vi "sub_rplidar_check.vi"(8 "error in (no error)":errorcluster) -> (0 "error out":errorcluster, 3 "ok":bool)   [LabVIEW 2019]
uses:
  Ctrl/rplidar_cmd.ctl
panel:
  out "read buffer":string
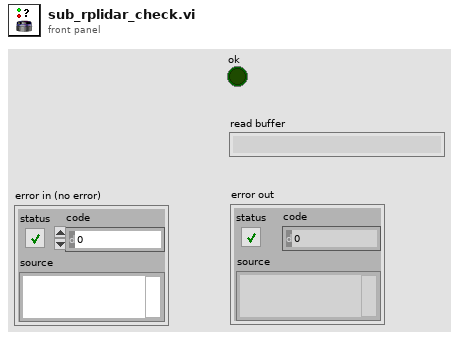
[diagram p1: front panel]
types:
  T1 = typedef "rplidar_cmd.ctl" = enum16{"init", "health", "spin", "scan", "read", "stop", "close"}
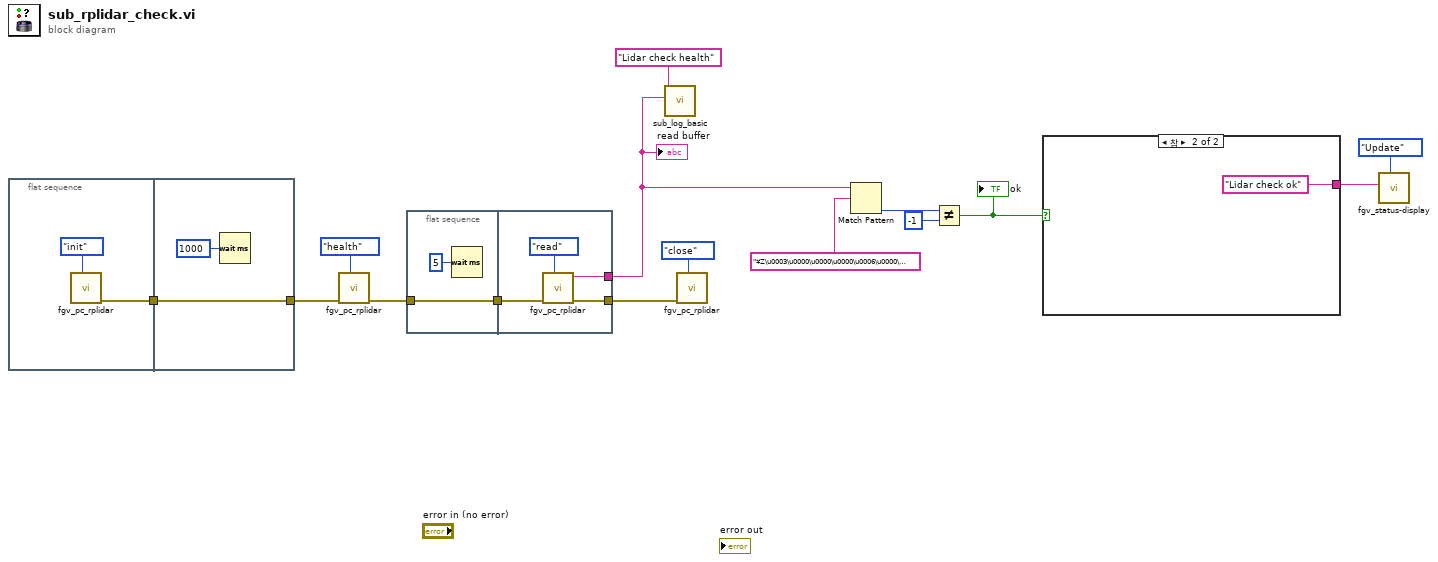
[diagram p0: block diagram]
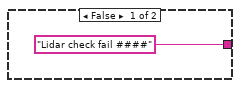
[diagram p2: hidden frame]
diagram:
  n1 = flat-sequence {
    tunnel: [w17] -> w12
    tunnel: [w19] -> w8
    tunnel: w12 -> [w19]
    frame #0 {
      n2 = call "fgv_pc_rplidar.vi"("cmd"=rplidar_cmd."init") -> ("error out"=w17:errorcluster)  [unwired: 8 in, 2 out]
    }
    frame #1 {
      n3 = Wait (ms)(milliseconds to wait=u32 1000) -> ()  [unwired: 1 out]
    }
  }
  n4 = call "fgv_pc_rplidar.vi"("cmd"=rplidar_cmd."health", "error in"=w8) -> ("error out"=w7:errorcluster)  [unwired: 7 in, 2 out]
  n5 = flat-sequence {
    tunnel: w7 -> [w21]
    tunnel: [w21] -> w6
    tunnel: [w24] -> w15
    tunnel: [w23] -> w4
    tunnel: w6 -> [w25]
    frame #0 {
      n6 = Wait (ms)(milliseconds to wait=u32 5) -> ()  [unwired: 1 out]
    }
    frame #1 {
      n7 = call "fgv_pc_rplidar.vi"("cmd"=rplidar_cmd."read", "error in"=w25) -> ("error out"=w24:errorcluster, "read buffer"=w23:string)  [unwired: 7 in, 1 out]
    }
  }
  n8 = call "sub_log_basic.vi"("desc"=w4, "Title"="Lidar check health") -> ()  [unwired: 9 in, 1 out]
  n9 = call "fgv_pc_rplidar.vi"("cmd"=rplidar_cmd."close", "error in"=w15) -> ()  [unwired: 7 in, 3 out]
  n10 = Match Pattern(string=w4, regular expression="¥Z\u0003\u0000\u0000\u0000\u0006\u0000\u0000\u0000") -> (offset past match=w2:i32)  [unwired: 1 in, 3 out]
  n11 = Not Equal?(x=w2, y=-1) -> (x != y?=w5:bool)
  "ok" <- w5
  n12 = case shown="참" w5 {
    tunnel: ["Lidar check fail ####" ("String in") "Lidar check ok" ("String in")] -> w13
    frame False {
    }
    frame True {
    }
  }
  n13 = call "fgv_status-display.vi"("Mode"=enum16{"Initial", "Update", "Clear"}."Update", "title"=w13) -> ()  [unwired: 9 in, 1 out]
  "read buffer" <- w4
